vi "Create New Page.vi"(8 "error in (no error)":errorcluster, 11 "xwpfWriter in":refnum<class "xwpfWriter.lvclass">) -> (0 "error out":errorcluster, 3 "xwpfWriter out":refnum<class "xwpfWriter.lvclass">)   [LabVIEW 2017, in "xwpfWriter.lvclass"]
uses:
  xwpfWriter.lvclass
  xwpfWriter.lvclass/xwpfWriter.ctl
  C:/Users/Neo/Desktop/Dev_Tools_BR/LabVIEW_NPOI/lib/NPOI 2.1.1/NPOI.OOXML.dll
  lib/NPOI 2.1.1/NPOI.OOXML.dll
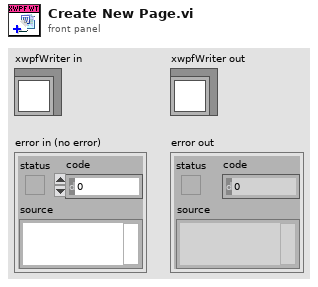
[diagram p1: front panel]
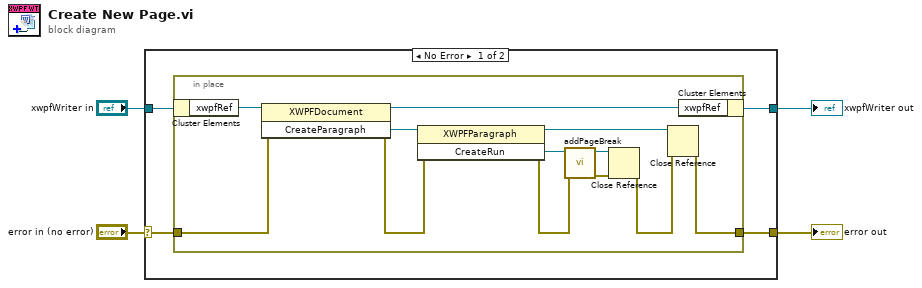
[diagram p0: block diagram]
diagram:
  n1 = case shown="No Error" "error in (no error)" {
    selector: "error in (no error)" -> [w6 w22]
    tunnel: [w5 w22] -> w3
    tunnel: [w7 w21] -> w1
    tunnel: "xwpfWriter in" -> [w8 w21]
    frame No Error {
      n2 = in-place {
        in-place-border: w6 -> [w10]
        in-place-border: [w9] -> w5
        n3 = in-place-cluster #1(w8) -> ("xwpfRef"=w20:refnum<k24>)
        n4 = invoke class="XWPFDocument" method="CreateParagraph"(reference=w20, error in=w10) -> (reference out=w18:refnum<k24>, error out=w11:errorcluster, "CreateParagraph"=w19:refnum<k24>)  [unwired: 1 in]
        n5 = invoke class="XWPFParagraph" method="CreateRun"(reference=w19, error in=w11) -> (reference out=w14:refnum<k24>, error out=w13:errorcluster, "CreateRun"=w17:refnum<k24>)  [unwired: 1 in]
        n6 = call "addPageBreak.vi"("error in (no error)"=w13, "WPFRun in"=w17) -> ("error out"=w16:errorcluster, "WPFRun out"=w15:refnum<k24>)  [unwired: 8 in]
        n7 = Close Reference(reference=w15, error in (no error)=w16) -> (error out=w12:errorcluster)
        n8 = Close Reference(reference=w14, error in (no error)=w12) -> (error out=w9:errorcluster)
        n9 = in-place-cluster #1("xwpfRef"=w18) -> (w7:refnum<class "xwpfWriter.lvclass">)
      }
    }
    frame Error {
    }
  }
  "error out" <- w3
  "xwpfWriter out" <- w1
